vi "FGV_OBJ_records_display.vi"(7 "options":T1, 8 "error_in":errorcluster, 11 "input":variant) -> (0 "error_out":errorcluster, 3 "output":variant)   [LabVIEW 2020]
uses:
  FGV_OBJ_records_display.ctl
  OBJ_all_info.ctl
  MAIN/OBJ_header_data_display.ctl
  MAIN/OBJ_measurement_status.ctl
  OBJ_references.ctl
  OBJ_history_display/FGV_OBJ_history_display.ctl
  tristate_indicator_OBJ_test/FGV_tristate_indicator_OBJ_test.ctl
  test_button/FGV_OBJ_test_button.ctl
  _misc/AULocalize/SubVIs/Get Localized Phrase Compact Interface 2D.vi
  _misc/AULocalize/SubVIs/Get Localized Phrase Compact Interface 1D.vi
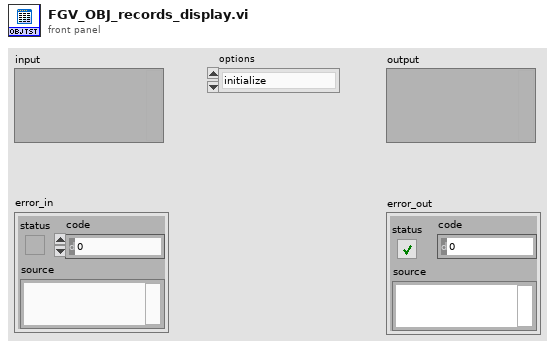
[diagram p1: front panel]
types:
  T1 = typedef "FGV_OBJ_records_display.ctl" = enum16{"initialize", "set_serial", "display_header", "display_results", "get_serial", "get_part_ID", "clear"}
  T2 = typedef "OBJ_references.ctl" = cluster{"front_panel_reference":refnum<vi>, "SQL_listbox_reference":refnum<vi>, "OBJ_header_data_display":refnum<vi>}
  T3 = typedef "OBJ_all_info.ctl" = cluster{"serial":string, "OBJ_header":T4, "ItemNames":string[][], "statuses":T5[], "OBJ_references":T2}
  T4 = typedef "OBJ_header_data_display.ctl" = cluster{"ID":string, "creation_time":string, "last_station":string, "last_status":string, "pinion_serial":string, "batch_code":string}
  T5 = typedef "OBJ_measurement_status.ctl" = enum16{"OK", "NOK"}
  T6 = typedef "FGV_OBJ_history_display.ctl" = enum16{"initialize", "add", "clear"}
  T7 = typedef "FGV_OBJ_test_button.ctl" = enum16{"initialize", "set_new_login", "set_message", "enable", "disable", "disable_gray", "translate", "set_scan_tooling", "get_scan_tooling"}
  T8 = typedef "FGV_tristate_indicator_OBJ_test.ctl" = enum16{"initialize", "tooling", "ready", "pending", "OK", "NOK", "part_NOK", "routing_NOK", "repeat_NOK", "timeout", "translate", "error"}
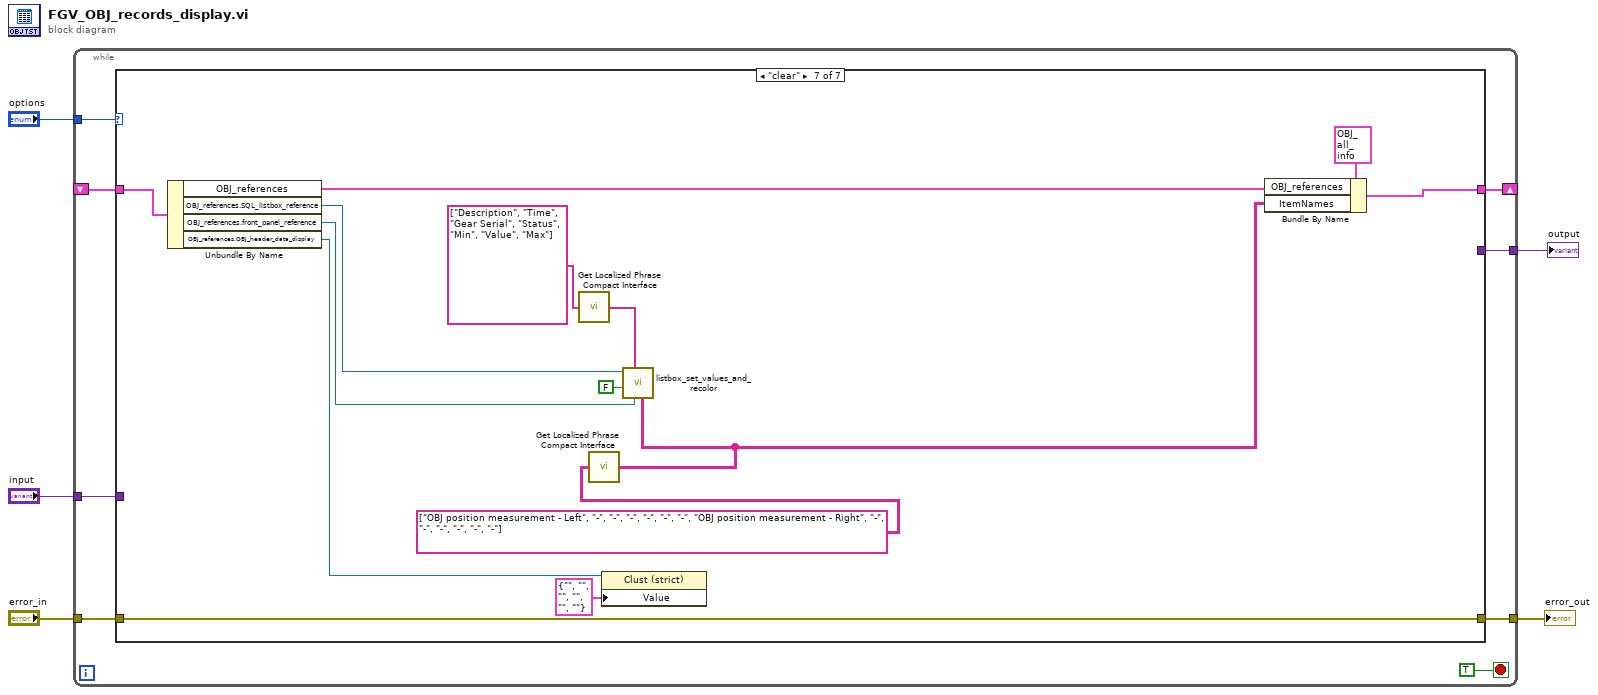
[diagram p0: block diagram]
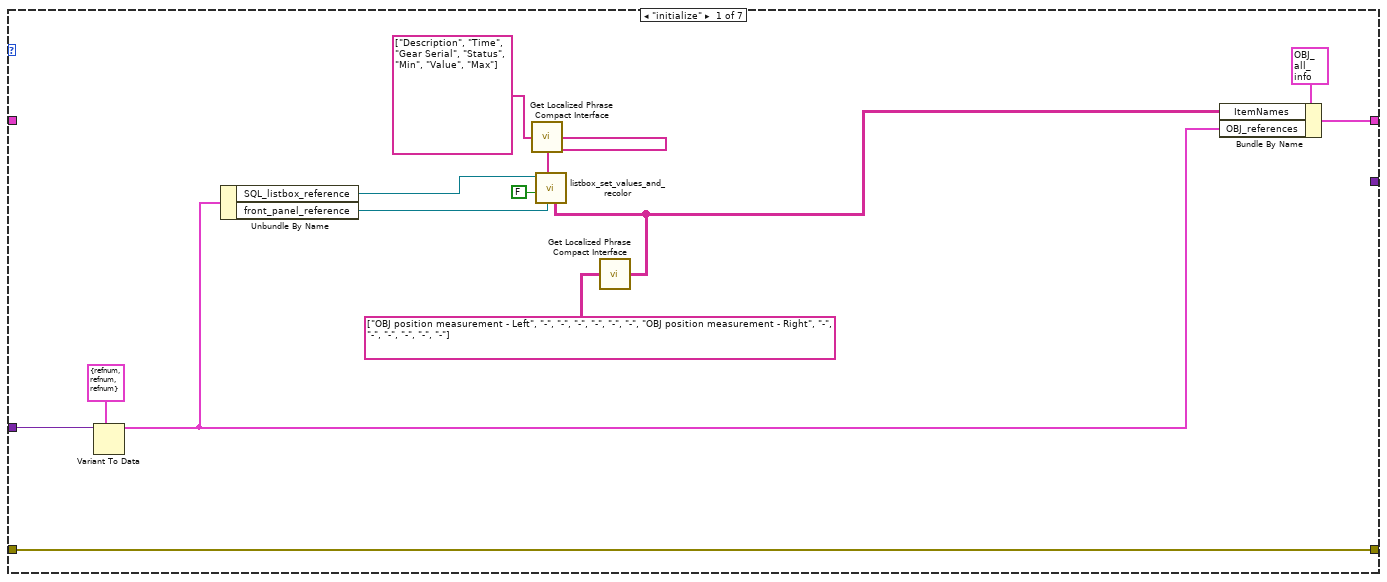
[diagram p2: hidden frame]
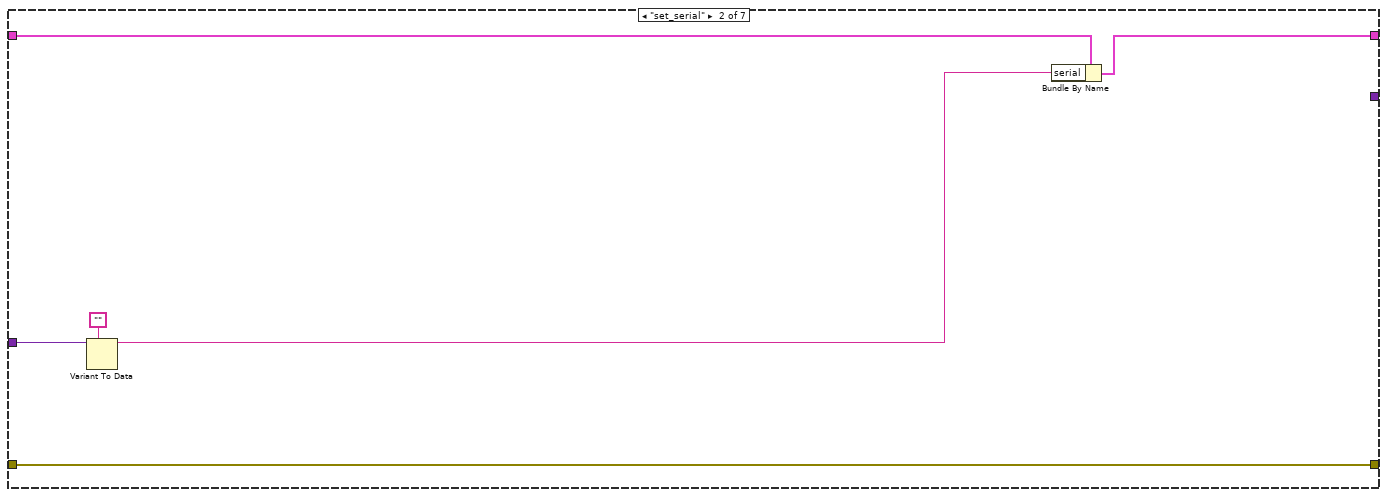
[diagram p3: hidden frame]
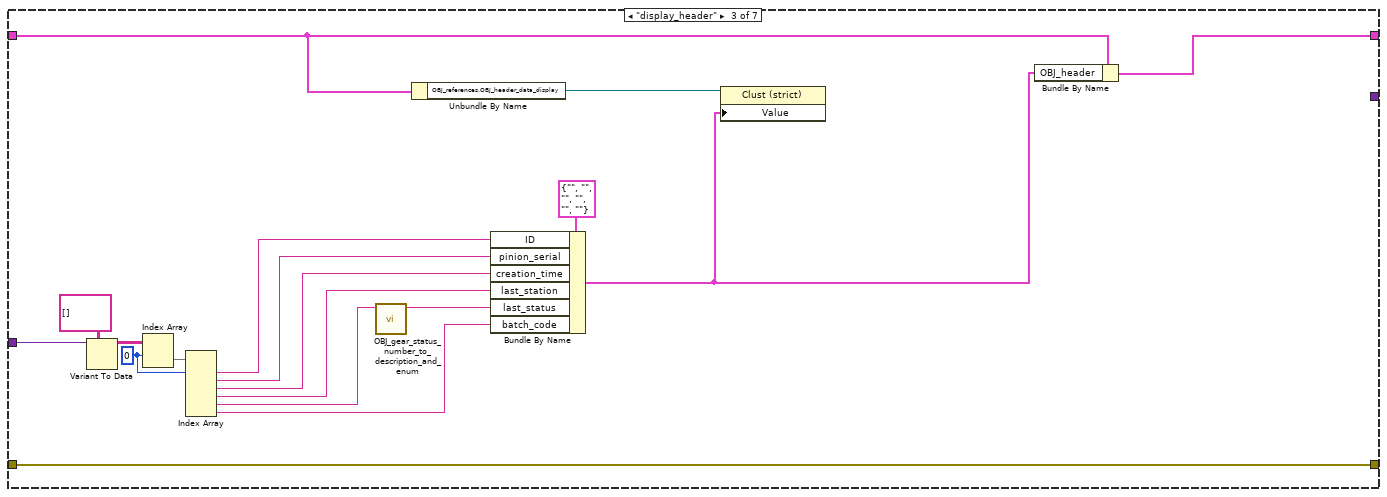
[diagram p4: hidden frame]
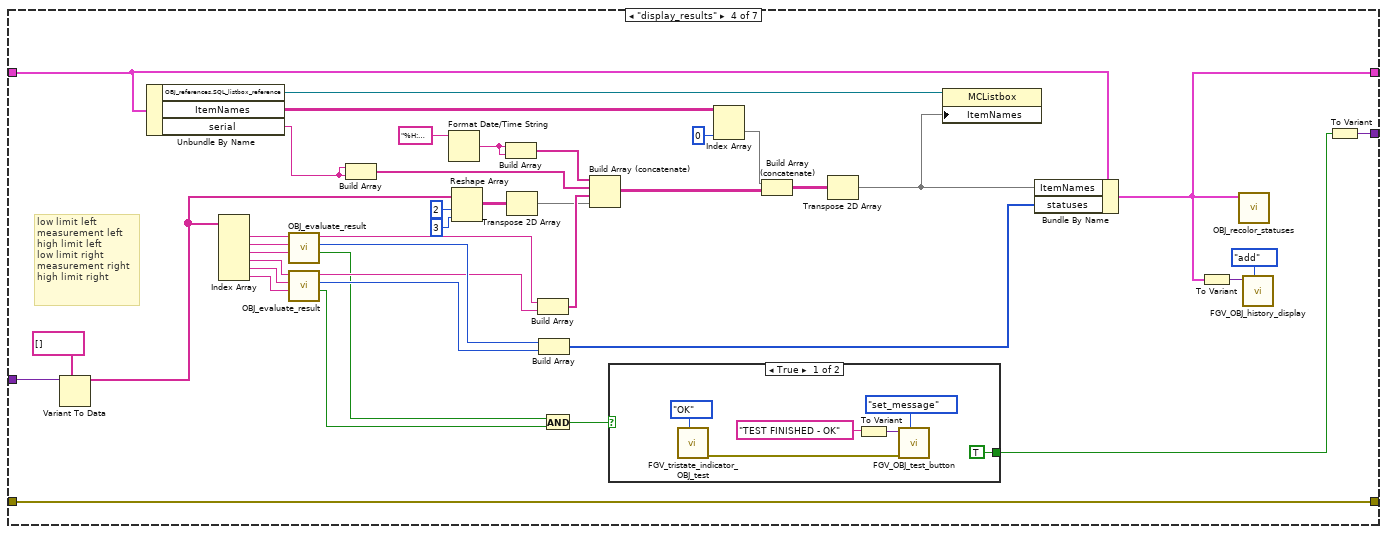
[diagram p5: hidden frame]
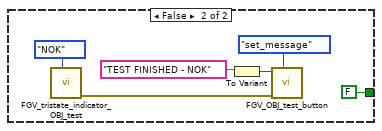
[diagram p6: hidden frame]
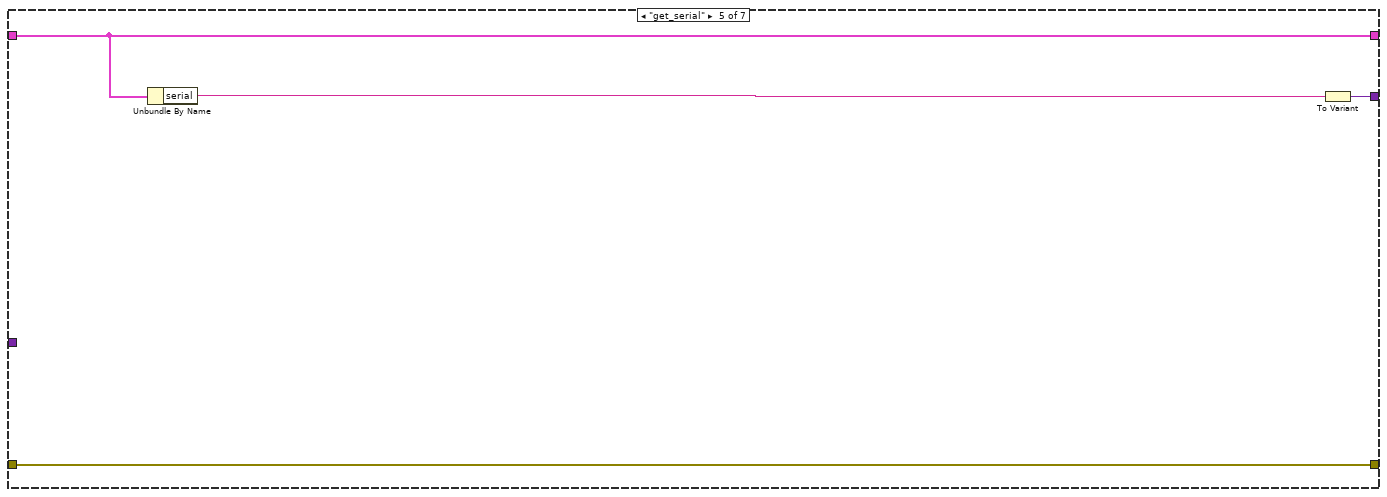
[diagram p7: hidden frame]
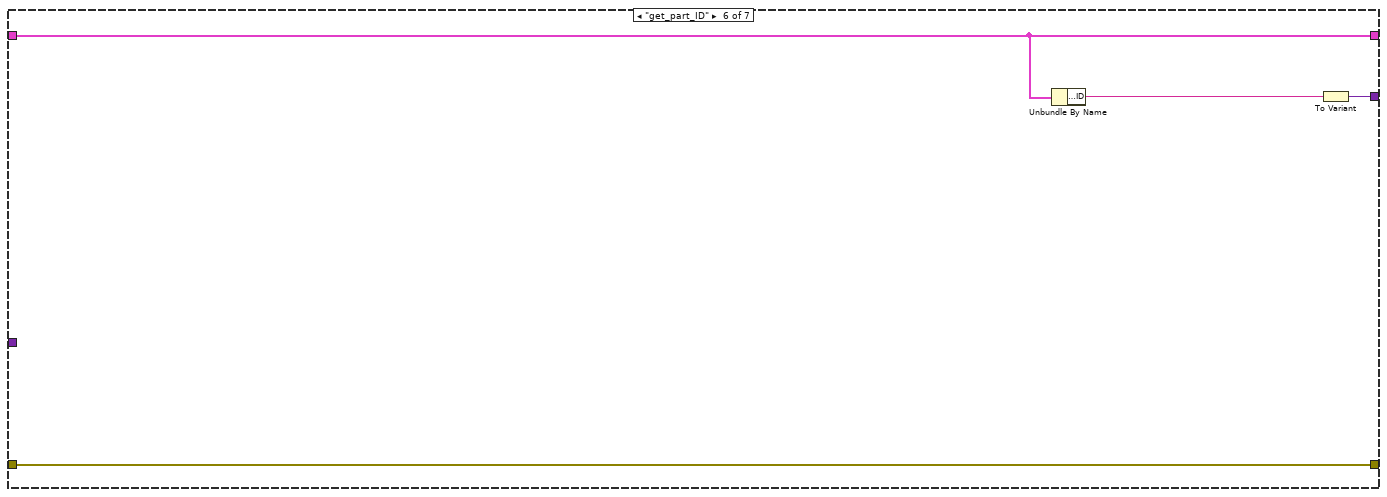
[diagram p8: hidden frame]
diagram:
  n1 = while {
    tunnel: "options" -> [w12]
    tunnel: [w11] -> w5
    tunnel: "error_in" -> [w10]
    shift-right: [w9] -> _
    shift-left: _ -> [w8]
    tunnel: "input" -> [w7]
    tunnel: [w6] -> w1
    stop <- TRUE stop-if-true
    n2 = case shown="\"clear\"" w12 {
      tunnel: [w26 w32 w50 w91 w107 w108 w125] -> w11
      tunnel: w10 -> [w26 w32 w50 w91 w107 w108 w125]
      tunnel: [w20 w31 w49 w63 w105 w111 w123] -> w9
      tunnel: w8 -> [_ w29 w40 w74 w105 w111 w124]
      tunnel: w7 -> [w24 w30 w48 w90 _ _ _]
      tunnel: [_ _ _ w61 w106 w110 _] -> w6
      frame "initialize" {
        n3 = Variant To Data(type=T2 {"front_panel_reference"=refnum, "SQL_listbox_reference"=refnum, "OBJ_header_data_display"=refnum} ("REWORK_references"), Variant=w24) -> (data=w21:T2)  [unwired: 1 in, 1 out]
        n4 = Unbundle By Name(w21) -> ("SQL_listbox_reference"=w22:refnum<vi>, "front_panel_reference"=w23:refnum<vi>)
        n5 = call-poly "Get Localized Phrase Compact Interface.vi"("Key"=string[] ["Description", "Time", "Gear Serial", "Status", "Min", "Value", "Max"] ("column_names")) -> ("Translated Phrase"=w15:string[])
        n6 = call-poly "Get Localized Phrase Compact Interface.vi"("Key"=string[][] [["OBJ position measurement - Left", "-", "-", "-", "-", "-", "-"], ["OBJ position measurement - Right", "-", "-", "-", "-", "-", "-"]] ("item_names")) -> ("Translated Phrase"=w14:string[][])
        n7 = call "listbox_set_values_and_recolor.vi"("item_names"=w14, "front_panel_reference"=w23, "column_names"=w15, "Autosize? (T)"=FALSE, "multicolumn_listbox_reference_in"=w22) -> ()  [unwired: 5 in, 2 out]
        n8 = Bundle By Name(cluster=T3 {"serial"="", "OBJ_header"={"ID"="", "creation_time"="", "last_station"="", "last_status"="", "pinion_serial"="", "batch_code"=""}, "ItemNames"=[], "statuses"=[], "OBJ_references"={"front_panel_reference"=refnum, "SQL_listbox_reference"=refnum, "OBJ_header_data_display"=refnum}} ("REPORT_all_info"), "ItemNames"=w14, "OBJ_references"=w21) -> (w20:T3)
      }
      frame "set_serial" {
        n9 = Variant To Data(type="", Variant=w30) -> (data=w27:string)  [unwired: 1 in, 1 out]
        n10 = Bundle By Name(cluster=w29, "serial"=w27) -> (w31:T3)
      }
      frame "display_header" {
        w44 = 0 ("index (row)")
        n11 = Variant To Data(type=string[][] [], Variant=w48) -> (data=w46:string[][])  [unwired: 1 in, 1 out]
        n12 = Index Array(array=w46, index (row)=w44) -> (element=w45:string[])  [unwired: 1 in]
        n13 = Index Array(array=w45, index #1=w44) -> (element #1=w42:string, element #2=w43:string, element #3=w41:string, element #4=w38:string, element #5=w36:string, element #6=w33:string)  [unwired: 5 in]
        n14 = call "OBJ_gear_status_number_to_description_and_enum.vi"("status_nmb"=w36) -> ("status_description"=w37:string)  [unwired: 9 in, 1 out]
        n15 = Unbundle By Name(w40) -> ("OBJ_references.OBJ_header_data_display"=w39:refnum<vi>)
        n16 = Bundle By Name(cluster=T4 {"ID"="", "creation_time"="", "last_station"="", "last_status"="", "pinion_serial"="", "batch_code"=""} ("REPORT_GEAR_header"), "ID"=w42, "pinion_serial"=w43, "creation_time"=w41, "last_station"=w38, "last_status"=w37, "batch_code"=w33) -> (w34:T4)
        n17 = property class="Clust (strict)"(reference=w39, "Value"=w34) -> ()  [unwired: 1 in, 2 out]
        n18 = Bundle By Name(cluster=w40, "OBJ_header"=w34) -> (w49:T3)
      }
      frame "display_results" {
        # "low limit left\nmeasurement left\nhigh limit left\nlow limit right\nmeasurement right\nhigh limit right"
        n19 = Variant To Data(type=string[] [], Variant=w90) -> (data=w85:string[])  [unwired: 1 in, 1 out]
        n20 = Unbundle By Name(w74) -> ("OBJ_references.SQL_listbox_reference"=w51:refnum<vi>, "ItemNames"=w72:string[][], "serial"=w53:string)
        n21 = Index Array(array=w85) -> (element #1=w88:string, element #2=w87:string, element #3=w86:string, element #4=w80:string, element #5=w79:string, element #6=w78:string)  [unwired: 6 in]
        n22 = call "OBJ_evaluate_result.vi"("high_limit"=w86, "measurement"=w87, "low_limit"=w88) -> ("OK?"=w67:bool, "status"=w81:T5, "status_string"=w82:string)  [unwired: 6 in]
        n23 = call "OBJ_evaluate_result.vi"("high_limit"=w78, "measurement"=w79, "low_limit"=w80) -> ("OK?"=w66:bool, "status"=w76:T5, "status_string"=w77:string)  [unwired: 6 in]
        n24 = Build Array(w53, w53) -> (w52:string[])
        n25 = Format Date/Time String(time format string (%c)="%H:%M:%S") -> (date/time string=w55:string)  [unwired: 2 in]
        n26 = Reshape Array(w85, 2 ("dimension size"), 3 ("dimension size")) -> (w69:string[][])
        n27 = Build Array(w55, w55) -> (w54:string[])
        n28 = Transpose 2D Array(2D array=w69) -> (transposed array=w68:string[][])
        n29 = Build Array(w82, w77) -> (w73:string[])
        n30 = Build Array(w81, w76) -> (w75:T5[])
        n31 = And(x=w67, y=w66) -> (x .and. y?=w65:bool)
        n32 = Build Array (concatenate)(w54, w52, w73, w68) -> (w59:string[][])
        n33 = case shown="True" w65 {
          tunnel: [TRUE FALSE] -> w60
          frame True {
            n34 = call "FGV_tristate_indicator_OBJ_test.vi"("options"=FGV_tristate_indicator_OBJ_test."OK") -> ("error_out"=w97:errorcluster)  [unwired: 10 in]
            n35 = To Variant(anything="TEST FINISHED - OK") -> (Variant=w96:variant)
            n36 = call "FGV_OBJ_test_button.vi"("options"=FGV_OBJ_test_button."set_message", "error_in"=w97, "input"=w96) -> ()  [unwired: 7 in, 2 out]
          }
          frame False {
            n37 = call "FGV_tristate_indicator_OBJ_test.vi"("options"=FGV_tristate_indicator_OBJ_test."NOK") -> ("error_out"=w103:errorcluster)  [unwired: 10 in]
            n38 = To Variant(anything="TEST FINISHED - NOK") -> (Variant=w102:variant)
            n39 = call "FGV_OBJ_test_button.vi"("options"=FGV_OBJ_test_button."set_message", "error_in"=w103, "input"=w102) -> ()  [unwired: 7 in, 2 out]
          }
        }
        n40 = Index Array(array=w72, index (col)=0 ("disabled index (col)")) -> (element=w70:string[])  [unwired: 1 in]
        n41 = Build Array (concatenate)(w70, w59) -> (w58:string[][])
        n42 = Transpose 2D Array(2D array=w58) -> (transposed array=w57:string[][])
        n43 = property class="MCListbox"(reference=w51, "ItemNames"=w57) -> ()  [unwired: 1 in, 2 out]
        n44 = Bundle By Name(cluster=w74, "ItemNames"=w57, "statuses"=w75) -> (w63:T3)
        n45 = To Variant(anything=w63) -> (Variant=w62:variant)
        n46 = call "OBJ_recolor_statuses.vi"("OBJ_all_info"=w63) -> ()  [unwired: 10 in, 1 out]
        n47 = call "FGV_OBJ_history_display.vi"("options"=FGV_OBJ_history_display."add", "input"=w62) -> ()  [unwired: 9 in, 1 out]
        n48 = To Variant(anything=w60) -> (Variant=w61:variant)
      }
      frame "get_serial" {
        n49 = Unbundle By Name(w105) -> ("serial"=w104:string)
        n50 = To Variant(anything=w104) -> (Variant=w106:variant)
      }
      frame "get_part_ID" {
        n51 = Unbundle By Name(w111) -> ("OBJ_header.ID"=w109:string)
        n52 = To Variant(anything=w109) -> (Variant=w110:variant)
      }
      frame "clear" {
        n53 = Unbundle By Name(w124) -> ("OBJ_references"=w114:T2, "OBJ_references.SQL_listbox_reference"=w121:refnum<vi>, "OBJ_references.front_panel_reference"=w120:refnum<vi>, "OBJ_references.OBJ_header_data_display"=w118:refnum<vi>)
        n54 = call-poly "Get Localized Phrase Compact Interface.vi"("Key"=string[] ["Description", "Time", "Gear Serial", "Status", "Min", "Value", "Max"] ("column_names")) -> ("Translated Phrase"=w112:string[])
        n55 = call-poly "Get Localized Phrase Compact Interface.vi"("Key"=string[][] [["OBJ position measurement - Left", "-", "-", "-", "-", "-", "-"], ["OBJ position measurement - Right", "-", "-", "-", "-", "-", "-"]] ("item_names")) -> ("Translated Phrase"=w115:string[][])
        n56 = property class="Clust (strict)"(reference=w118, "Value"=T4 {"ID"="", "creation_time"="", "last_station"="", "last_status"="", "pinion_serial"="", "batch_code"=""}) -> ()  [unwired: 1 in, 2 out]
        n57 = call "listbox_set_values_and_recolor.vi"("item_names"=w115, "front_panel_reference"=w120, "column_names"=w112, "Autosize? (T)"=FALSE, "multicolumn_listbox_reference_in"=w121) -> ()  [unwired: 5 in, 2 out]
        n58 = Bundle By Name(cluster=T3 {"serial"="", "OBJ_header"={"ID"="", "creation_time"="", "last_station"="", "last_status"="", "pinion_serial"="", "batch_code"=""}, "ItemNames"=[], "statuses"=[], "OBJ_references"={"front_panel_reference"=refnum, "SQL_listbox_reference"=refnum, "OBJ_header_data_display"=refnum}} ("REPORT_all_info"), "OBJ_references"=w114, "ItemNames"=w115) -> (w123:T3)
      }
    }
  }
  "error_out" <- w5
  "output" <- w1
